vi "test-ramsete.vi"(8 "error in (no error)":errorcluster) -> (0 "error out":errorcluster, 3 "AtReference End":bool)   [LabVIEW 2019]
uses:
  <vilib>/Rock Robotics/WPI/ThirdParty/JAS_Junk/TrajLib/CHASSIS_SPEEDS.ctl
  <vilib>/Rock Robotics/WPI/ThirdParty/JAS_Junk/TrajLib/POSE2D.ctl
  <vilib>/Rock Robotics/WPI/ThirdParty/JAS_Junk/TrajLib/TRANSLATION2D.ctl
  <vilib>/Rock Robotics/WPI/ThirdParty/JAS_Junk/TrajLib/ROTATION2D.ctl
  <vilib>/Rock Robotics/WPI/ThirdParty/JAS_Junk/TrajLib/TRAJ_STATE.ctl
  <vilib>/Rock Robotics/WPI/ThirdParty/JAS_Junk/TrajLib/TRAJECTORY.ctl
  <vilib>/Rock Robotics/WPI/ThirdParty/JAS_Junk/TrajLib/Conv_Inches_Meters.vi
  <vilib>/Rock Robotics/WPI/ThirdParty/JAS_Junk/TrajLib/Rotation2d_CreateAngle.vi
  <vilib>/Rock Robotics/WPI/ThirdParty/JAS_Junk/TrajLib/Translation2d_Create.vi
  <vilib>/Rock Robotics/WPI/ThirdParty/JAS_Junk/TrajLib/Trajectory_Library.lvlib
panel:
  out "poseError":T1={"TRANSLATION"={"X"=0.0, "Y"=0.0}, "ROTATION"={"VALUE"=0.0, "COS"=1.0, "SIN"=0.0}} {"ROTATION"."SIN" format="%13.4f"; "ROTATION"."COS" format="%13.4f"; "ROTATION"."VALUE" format="%13.4f"; "TRANSLATION"."Y" format="%14.3f"; "TRANSLATION"."X" format="%14.3f"}
  out "AtReference":bool
  out "end POSe":T1 {"ROTATION"."SIN" format="%13.4f"; "ROTATION"."COS" format="%13.4f"; "ROTATION"."VALUE" format="%13.4f"; "TRANSLATION"."Y" format="%14.3f"; "TRANSLATION"."X" format="%14.3f"}
  out "TRAJECTORY":T4 {"States"."POSE"."ROTATION"."SIN" format="%13.4f"; "States"."POSE"."ROTATION"."COS" format="%13.4f"; "States"."POSE"."ROTATION"."VALUE" format="%13.4f"; "States"."POSE"."TRANSLATION"."Y" format="%14.3f"; "States"."POSE"."TRANSLATION"."X" format="%14.3f"; "TotalTImeSecs" format="%20.3f"}
  out "OutputTRAJ_STATE":T5={"TimeSeconds"=0.0, "Velocity"=0.0, "Acceleration"=0.0, "POSE"={"TRANSLATION"={"X"=0.0, "Y"=0.0}, "ROTATION"={"VALUE"=0.0, "COS"=1.0, "SIN"=0.0}}, "Curvature"=0.0} {"POSE"."ROTATION"."SIN" format="%13.4f"; "POSE"."ROTATION"."COS" format="%13.4f"; "POSE"."ROTATION"."VALUE" format="%13.4f"; "POSE"."TRANSLATION"."Y" format="%14.3f"; "POSE"."TRANSLATION"."X" format="%14.3f"}
  out "Integer":i32
  out "UpdatedPose":T1 {"ROTATION"."SIN" format="%13.4f"; "ROTATION"."COS" format="%13.4f"; "ROTATION"."VALUE" format="%13.4f"; "TRANSLATION"."Y" format="%14.3f"; "TRANSLATION"."X" format="%14.3f"}
  out "CHASSIS Speeds":T6 {"vOmega" format="%10.3f"; "vY" format="%10.3f"; "vX" format="%10.3f"}
  out "Samp-int":i32
  out "Samp-real":dbl
  # "Ramsete"
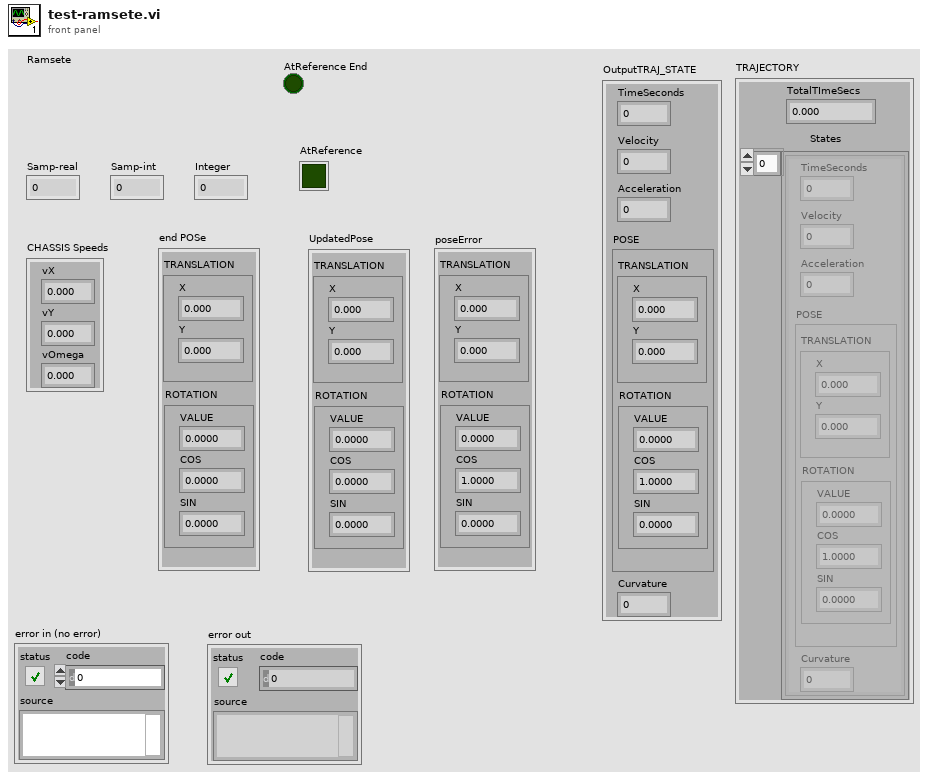
[diagram p1: front panel]
types:
  T1 = typedef "Trajectory_Library.lvlib/POSE2D.ctl" = cluster{"TRANSLATION":T2, "ROTATION":T3}
  T2 = typedef "Trajectory_Library.lvlib/TRANSLATION2D.ctl" = cluster{"X":dbl, "Y":dbl}
  T3 = typedef "Trajectory_Library.lvlib/ROTATION2D.ctl" = cluster{"VALUE":dbl, "COS":dbl, "SIN":dbl}
  T4 = typedef "Trajectory_Library.lvlib/TRAJECTORY.ctl" = cluster{"TotalTImeSecs":dbl, "States":T5[]}
  T5 = typedef "Trajectory_Library.lvlib/TRAJ_STATE.ctl" = cluster{"TimeSeconds":dbl, "Velocity":dbl, "Acceleration":dbl, "POSE":T1, "Curvature":dbl}
  T6 = typedef "Trajectory_Library.lvlib/CHASSIS_SPEEDS.ctl" = cluster{"vX":dbl, "vY":dbl, "vOmega":dbl}
  T7 = typedef "Trajectory_Library.lvlib/TRAJ_CONFIG.ctl" = cluster{"MaxVelocity":dbl, "Max Acceleration":dbl, "StartVelocity":dbl, "End Velocity":dbl, "Reversed":bool, "DiffDrKineConstntDefined":bool, "CentAcellConstntDefined":bool, "DiffDrVoltConstntDefined":bool, "DIFF_DRIVE_KINE_CONSTRAINT":T8, "CENTRIPETAL_ACCEL_CONSTRAINT":T10, "SwerveDrKineConstntDefined":bool, "SWERVE_DRIVE_KINE_CONSTRAINT":T11, "DIFF_DRIVE_VOLTAGE_CONSTRAINT":T14, "MECANUM_DRIVE_KINE_CONSTRAINT":T16, "MecanumDrKineConstntDefined":bool}
  T8 = typedef "Trajectory_Library.lvlib/TRAJ_CONSTRAINT_DIIF_DRIVE_KINEMATICS.ctl" = cluster{"Max Speed (M/S)":dbl, "DIFF_DRIVE_KINEMATICS":T9, "Max Accel (M/S2)":dbl}
  T9 = typedef "Trajectory_Library.lvlib/DIFF_DRIVE_KINEMATICS.ctl" = cluster{"TrackWidth_Meters":dbl}
  T10 = typedef "Trajectory_Library.lvlib/TRAJ_CONSTRAINT_CENTRIPETAL_ACCEL.ctl" = cluster{"Max Cent Accel":dbl}
  T11 = typedef "Trajectory_Library.lvlib/TRAJ_CONSTRAINT_SWERVE_DRIVE_KINEMATICS.ctl" = cluster{"Max Speed (M/S)":dbl, "SwerveKinematics":T12}
  T12 = typedef "Trajectory_Library.lvlib/SWERVE_DRIVE_KINEMATICS.ctl" = cluster{"NumModules":i32, "InverseKinematics":T13, "ForwardKinematics":T13, "Modules":T2[], "PrevCoR":T2}
  T13 = typedef "NI_Matrix.lvlib/RealMatrix.ctl" = dbl[][]
  T14 = typedef "Trajectory_Library.lvlib/TRAJ_CONSTRAINT_DIIF_DRIVE_VOLTAGE.ctl" = cluster{"Max Voltage":dbl, "DIFF_DRIVE_KINEMATICS":T9, "SIMPLE_MOTOR_FF":T15}
  T15 = typedef "Trajectory_Library.lvlib/SIMPLE_MOTOR_FF.ctl" = cluster{"Ks":dbl, "Kv":dbl, "Ka":dbl}
  T16 = typedef "Trajectory_Library.lvlib/TRAJ_CONSTRAINT_MECA_DRIVE_KINEMATICS.ctl" = cluster{"Max Speed (M/S)":dbl, "MECA_DRIVE_KINEMATICS":T17}
  T17 = typedef "Trajectory_Library.lvlib/MECA_DRIVE_KINEMATICS.ctl" = cluster{"FrontLeft":T2, "FrontRight":T2, "RearLeft":T2, "RearRight":T2, "InverseKinematics":T13, "ForwardKinematics":T13, "PrevCoR":T2}
  T18 = typedef "Trajectory_Library.lvlib/RAMSETE.ctl" = cluster{"B":dbl, "Zeta":dbl, "poseTolerance":T1, "poseError":T1, "Enabled":bool}
  T19 = typedef "Trajectory_Library.lvlib/TWIST2D.ctl" = cluster{"dX":dbl, "dY":dbl, "dTHETA":dbl}
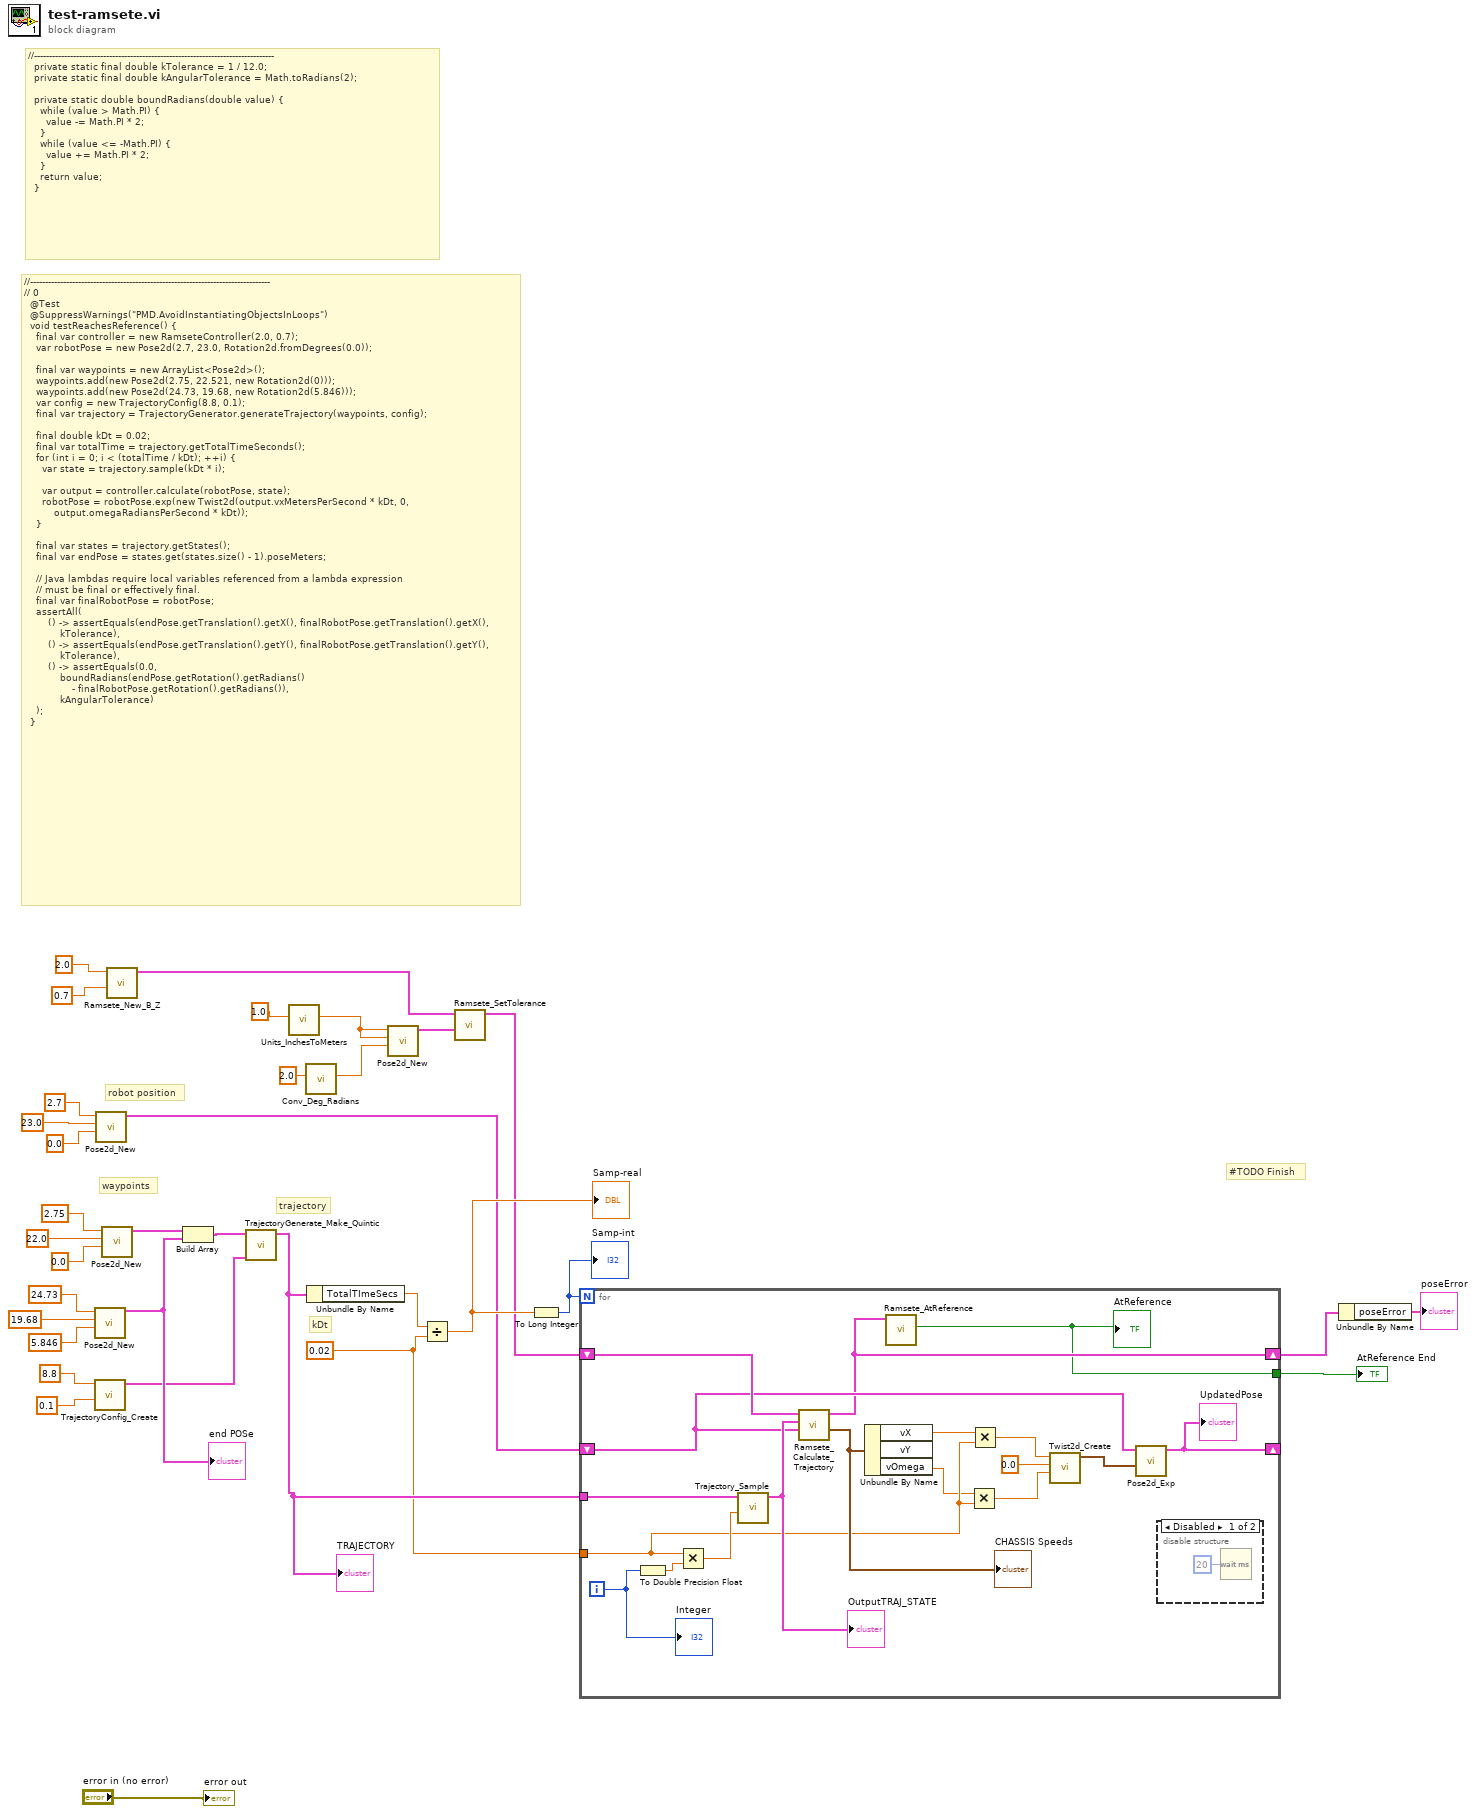
[diagram p0: block diagram]
diagram:
  w12 = 0.02
  # "#TODO Finish"
  # "kDt"
  # "trajectory"
  # "waypoints"
  # "robot position"
  # "//--------------------------------------------------------------------------------\n  private static final double kTolerance = 1 / 12.0;\n  private static final double kAngularTolerance = Math.toRadians(2);\n\n  private static double boundRadians(double value) {\n    while (value > Math.PI) {\n      value -= Math.PI * 2;\n    }\n    while (value <= -Math.PI) {\n      value += Math.PI * 2;\n    }\n    return value;\n  }"
  # "//--------------------------------------------------------------------------------\n// 0\n  @Test\n  @SuppressWarnings(\"PMD.AvoidInstantiatingObjectsInLoops\")\n  void testReachesReference() {\n    final var controller = new RamseteController(2.0, 0.7);\n    var robotPose = new Pose2d(2.7, 23.0, Rotation2d.fromDegrees(0.0));\n\n    final var waypoints = new ArrayList<Pose2d>();\n    waypoints.add(new Pose2d(2.75, 22.521, new Rotation2d(0)));\n    waypoints.add(new Pose2d(24.73, 19.68, new Rotation2d(5.846)));\n    var config = new TrajectoryConfig(8.8, 0.1);\n    final var trajectory = TrajectoryGenerator.generateTrajectory(waypoints, config);\n\n    final double kDt = 0.02;\n    final var totalTime = trajectory.getTotalTimeSeconds();\n    for (int i = 0; i < (totalTime / kDt); ++i) {\n      var state = trajectory.sample(kDt * i);\n\n      var output = controller.calculate(robotPose, state);\n      robotPose = robotPose.exp(new Twist2d(output.vxMetersPerSecond * kDt, 0,\n          output.omegaRadiansPerSecond * kDt));\n    }\n\n    final var states = trajectory.getStates();\n    final var endPose = states.get(states.size() - 1).poseMeters;\n\n    // Java lambdas require local variables referenced from a lambda expression\n    // must be final or effectively final.\n    final var finalRobotPose = robotPose;\n    assertAll(\n        () -> assertEquals(endPose.getTranslation().getX(), finalRobotPose.getTranslation().getX(),\n            kTolerance),\n        () -> assertEquals(endPose.getTranslation().getY(), finalRobotPose.getTranslation().getY(),\n            kTolerance),\n        () -> assertEquals(0.0,\n            boundRadians(endPose.getRotation().getRadians()\n                - finalRobotPose.getRotation().getRadians()),\n            kAngularTolerance)\n    );\n  }"
  n1 = call <vilib>:"Pose2d_New.vi"("Heading"=5.846, "Y"=19.68, "X"=24.73) -> ("out POSe"=w22:T1)  [unwired: 8 in]
  "end POSe" <- w22
  n2 = call <vilib>:"TrajectoryConfig_Create.vi"("MaxAcceleration"=0.1, "MaxVelocity"=8.8) -> ("TRAJECTORY_CONFIG"=w18:T7)  [unwired: 9 in]
  n3 = call <vilib>:"Pose2d_New.vi"("Heading"=0.0, "Y"=23.0, "X"=2.7) -> ("out POSe"=w13:T1)  [unwired: 8 in]
  n4 = call <vilib>:"Pose2d_New.vi"("Heading"=0.0, "Y"=22.0, "X"=2.75) -> ("out POSe"=w23:T1)  [unwired: 8 in]
  n5 = call <vilib>:"Ramsete_New_B_Z.vi"("Zeta"=0.7, "B"=2.0) -> ("outRAMSETE"=w7:T18)  [unwired: 9 in]
  n6 = Build Array(w23, w22) -> (w19:T1[])
  n7 = call <vilib>:"TrajectoryGenerate_Make_Quintic.vi"("traj_config"=w18, "waypointPOSE"=w19) -> ("TRAJECTORY"=w14:T4)  [unwired: 8 in, 1 out]
  "TRAJECTORY" <- w14
  n8 = call <vilib>:"Units_InchesToMeters.vi"("Inches"=1.0 ("x")) -> ("Meters"=w4:dbl)  [unwired: 10 in]
  n9 = call <vilib>:"Conv_Deg_Radians.vi"("Degress"=2.0) -> ("Radians"=w10:dbl)  [unwired: 10 in]
  n10 = Unbundle By Name(w14) -> ("TotalTImeSecs"=w17:dbl)
  n11 = call <vilib>:"Pose2d_New.vi"("Heading"=w10, "Y"=w4, "X"=w4) -> ("out POSe"=w9:T1)  [unwired: 8 in]
  n12 = Divide(x=w17, y=w12) -> (x/y=w15:dbl)
  "Samp-real" <- w15
  n13 = call <vilib>:"Ramsete_SetTolerance.vi"("tolerancePose"=w9, "inRAMSETE"=w7) -> ("outRAMSETE"=w8:T18)  [unwired: 9 in]
  n14 = To Long Integer(number=w15) -> (32bit integer=w16:i32)
  "Samp-int" <- w16
  n15 = for {
    N: w16 -> [_]
    tunnel: w12 -> [w43]
    tunnel: w14 -> [w50]
    shift-right: [w37] -> _
    shift-left: w13 -> [w39]
    shift-right: [w36] -> w2
    shift-left: w8 -> [w48]
    tunnel: [w35] -> w6
    i -> [w51]
    n16 = To Double Precision Float(number=w51) -> (double precision float=w52:dbl)
    n17 = Multiply(x=w43, y=w52) -> (x*y=w49:dbl)
    n18 = call <vilib>:"Trajectory_Sample.vi"("Time"=w49, "InputTRAJECTORY"=w50) -> ("OutputTRAJ_STATE"=w47:T5)  [unwired: 9 in]
    "OutputTRAJ_STATE" <- w47
    n19 = call <vilib>:"Ramsete_Calculate_Trajectory.vi"("CurrentPOSE"=w39, "TRAJ_STATE"=w47, "inRAMSETE"=w48) -> ("CHASSIS Speeds"=w46:T6, "outRAMSETE"=w36:T18)  [unwired: 7 in]
    "CHASSIS Speeds" <- w46
    n20 = Unbundle By Name(w46) -> ("vX"=w45:dbl, "vOmega"=w42:dbl)  [unwired: 1 out]
    n21 = call <vilib>:"Ramsete_AtReference.vi"("RAMSETE"=w36) -> ("AtReference"=w35:bool)  [unwired: 10 in]
    "AtReference" <- w35
    n22 = Multiply(x=w42, y=w43) -> (x*y=w40:dbl)
    n23 = Multiply(x=w45, y=w43) -> (x*y=w44:dbl)
    n24 = call <vilib>:"Twist2d_Create.vi"("dTHETA"=w40, "dY"=0.0, "dX"=w44) -> ("TWIST"=w38:T19)  [unwired: 8 in]
    n25 = call <vilib>:"Pose2d_Exp.vi"("TWIST"=w38, "POSE"=w39) -> ("UpdatedPose"=w37:T1)  [unwired: 9 in]
    "UpdatedPose" <- w37
    n26 = disable-structure shown="Disabled" {
      frame Disabled {
        n27 = Wait (ms)(milliseconds to wait=u32 20) -> ()  [unwired: 1 out]
      }
      frame Enabled {
      }
    }
    "Integer" <- w51
  }
  "AtReference End" <- w6
  n28 = Unbundle By Name(w2) -> ("poseError"=→"poseError":T1)
  "error out" <- "error in (no error)"
